vi "KH Control.vi"(6 "Radio Buttons":T1(radio), 8 "error in":errorcluster, 11 "Channel Setting":T7=[{"Channel"=enum."Channel 1", "Gain"=enum."10x", "Shunt Resistor"=enum."Open", "Input Config"=enum."Ground"}, {"Channel"=enum."Channel 2", "Gain"=enum."10x", "Shunt Resistor"=enum."Open", "Input Config"=enum."Ground"}, {"Channel"=enum."Channel 3", "Gain"=enum."10x", "Shunt Resistor"=enum."Open", "Input Config"=enum."Ground"}, {"Channel"=enum."Channel 4", "Gain"=enum."10x", "Shunt Resistor"=enum."Open", "Input Config"=enum."Ground"}, {"Channel"=enum."Channel 5", "Gain"=enum."10x", "Shunt Resistor"=enum."Open", "Input Config"=enum."Ground"}, {"Channel"=enum."Channel 6", "Gain"=enum."10x", "Shunt Resistor"=enum."Open", "Input Config"=enum."Ground"}, {"Channel"=enum."Channel 7", "Gain"=enum."10x", "Shunt Resistor"=enum."Open", "Input Config"=enum."Ground"}, {"Channel"=enum."Channel 8", "Gain"=enum."10x", "Shunt Resistor"=enum."Open", "Input Config"=enum."Ground"}]) -> (0 "error out":errorcluster={"status"=FALSE, "code"=1073676294, "source"="VISA Read in KH7008.lvclass:KH7008 COM.vi->KH7008.lvclass:KH7008 Set All.vi->KH7008.lvclass:KH Control.vi"}, 3 "Channel Settings Used":T2[](array[typedef])=[{"Channel"=enum."Channel 1", "Gain"=enum."10x", "Shunt Resistor"=enum."Open", "Input Config"=enum."Ground"}, {"Channel"=enum."Channel 2", "Gain"=enum."10x", "Shunt Resistor"=enum."Open", "Input Config"=enum."Ground"}, {"Channel"=enum."Channel 3", "Gain"=enum."10x", "Shunt Resistor"=enum."Open", "Input Config"=enum."Ground"}, {"Channel"=enum."Channel 4", "Gain"=enum."10x", "Shunt Resistor"=enum."Open", "Input Config"=enum."Ground"}, {"Channel"=enum."Channel 5", "Gain"=enum."10x", "Shunt Resistor"=enum."Open", "Input Config"=enum."Ground"}, {"Channel"=enum."Channel 6", "Gain"=enum."10x", "Shunt Resistor"=enum."Open", "Input Config"=enum."Ground"}, {"Channel"=enum."Channel 7", "Gain"=enum."10x", "Shunt Resistor"=enum."Open", "Input Config"=enum."Ground"}, {"Channel"=enum."Channel 8", "Gain"=enum."10x", "Shunt Resistor"=enum."Open", "Input Config"=enum."Ground"}])   [LabVIEW 2016, in "KH7008.lvclass"]
uses:
  KH7008.lvclass
  typedefs/KH_control_array.ctl
  typedefs/KH_control.ctl
  typedefs/Channel-Enum.ctl
  typedefs/Gain-Enum.ctl
  typedefs/Shunt-Enum.ctl
  typedefs/Input Configuration-Enum.ctl
  typedefs/SetAll-Cluster.ctl
  typedefs/Filter-Enum.ctl
  typedefs/Coupling-Enum.ctl
  <vilib>/MakerHub/Toolbox/LMH-Toolbox.lvlib
panel:
  in  "VISA Refnum in":refnum<visa-resource-name>="COM3"
  # "Measure Current: Current, Shunt Resistor: 50kOhm\nMeasure Voltage: Voltage, Shunt Resistor: Open\nApplying Gate: Current, Shunt Resistor: 50kOhm\n                      Open all the unused gate\n\n1. Create a copy of drivers under C:\\Krohn-Hite 7008\\Drivers if there is none. \n2. In device manager browse the driver for Krohn-Hite \n\nWarning: repeated channels will cause false reading in the lock-in"
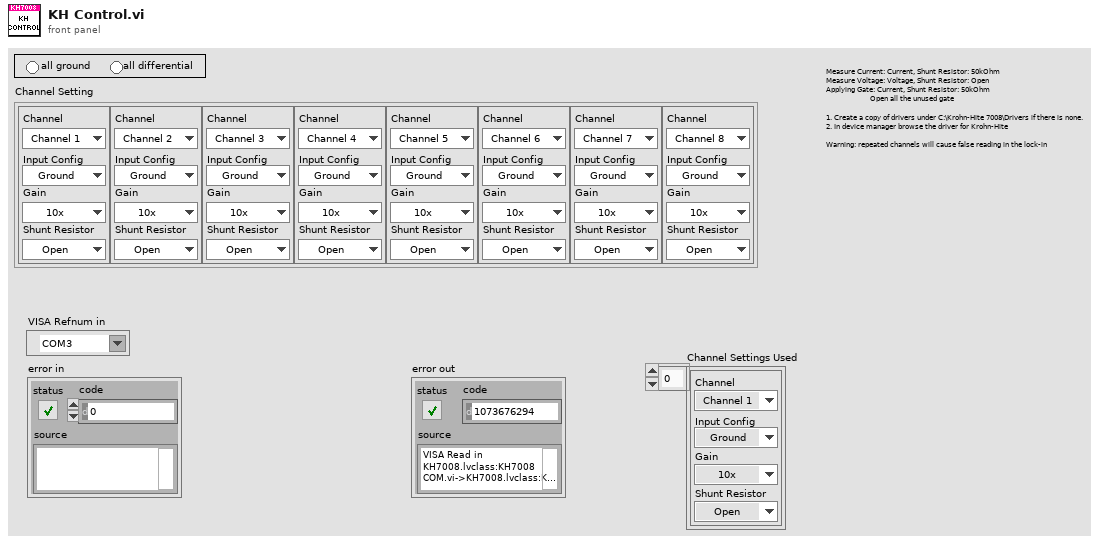
[diagram p1: front panel]
types:
  T1 = enum32{"No Selection", "all ground", "all differential"}
  T2 = typedef "KH7008.lvclass/KH_control.ctl" = cluster{"Channel":T3, "Gain":T4, "Shunt Resistor":T5, "Input Config":T6}
  T3 = typedef "KH7008.lvclass/Channel-Enum.ctl" = enum16{"Channel 1", "Channel 2", "Channel 3", "Channel 4", "Channel 5", "Channel 6", "Channel 7", "Channel 8"}
  T4 = typedef "KH7008.lvclass/Gain-Enum.ctl" = enum16{"1x", "10x", "100x", "1000x"}
  T5 = typedef "KH7008.lvclass/Shunt-Enum.ctl" = enum16{"Open", "50 Ohms", "500 Ohms", "5k Ohms", "50k Ohms"}
  T6 = typedef "KH7008.lvclass/Input Configuration-Enum.ctl" = enum16{"Ground", "SE+ (-gnd)", "SE- (+gnd)", "Differential"}
  T7 = typedef "KH7008.lvclass/KH_control_array.ctl" = T2[]
  T8 = typedef "KH7008.lvclass/Coupling-Enum.ctl" = enum16{"AC", "DC"}
  T9 = typedef "KH7008.lvclass/Filter-Enum.ctl" = enum16{"OFF", "ON"}
  T10 = typedef "KH7008.lvclass/SetAll-Cluster.ctl" = cluster{"Channel":T3, "Gain":T4, "Bandwidth Filter":T9, "Shunt Resistor":T5, "Coupling":T8, "Input Configuration":T6}
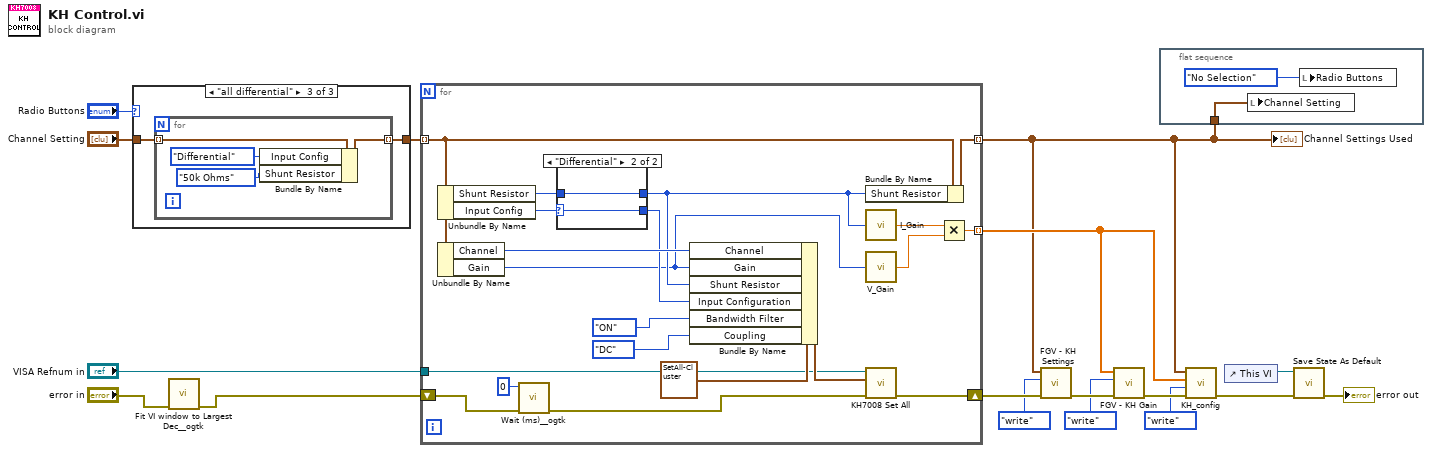
[diagram p0: block diagram]
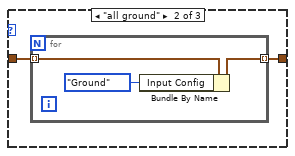
[diagram p3: hidden frame]
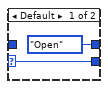
[diagram p4: hidden frame]
diagram:
  n1 = case shown="\"all differential\"" "Radio Buttons" {
    tunnel: [w18 w20 w25] -> w8
    tunnel: "Channel Setting" -> [w18 w19 w24]
    frame "No Selection", Default {
    }
    frame "all ground" {
      n2 = for {
        tunnel: w19 -> [w23] mode=indexing
        tunnel: [w22] -> w20 mode=indexing
        n3 = Bundle By Name(cluster=w23, "Input Config"=Input_Configuration-Enum."Ground") -> (w22:T2)
      }
    }
    frame "all differential" {
      n4 = for {
        tunnel: w24 -> [w29] mode=indexing
        tunnel: [w28] -> w25 mode=indexing
        n5 = Bundle By Name(cluster=w29, "Input Config"=Input_Configuration-Enum."Differential", "Shunt Resistor"=Shunt-Enum."50k Ohms") -> (w28:T2)
      }
    }
  }
  n6 = call <userlib>:"Fit VI window to Largest Dec__ogtk.vi"("error in (no error)"="error in") -> ("error out"=w3:errorcluster)  [unwired: 5 in, 1 out]
  n7 = for {
    tunnel: w8 -> [w34] mode=indexing
    tunnel: [w49] -> w5 mode=indexing
    shift-right: [w47] -> w13
    shift-left: w3 -> [w48]
    tunnel: [w41] -> w1 mode=indexing
    tunnel: "VISA Refnum in" -> [w40]
    n8 = Unbundle By Name(w34) -> ("Shunt Resistor"=w36:T5, "Input Config"=w35:T6)
    n9 = Unbundle By Name(w34) -> ("Channel"=w39:T3, "Gain"=w30:T4)
    n10 = call <userlib>:"Wait (ms)__ogtk.vi"("error in (no error)"=w48, "milliseconds to wait"=u32 0) -> ("error out"=w46:errorcluster)  [unwired: 8 in, 1 out]
    n11 = case shown="\"Differential\"" w35 {
      selector: w35 -> [w50 w52]
      tunnel: [Shunt-Enum."Open" ("f") w53] -> w33
      tunnel: w36 -> [_ w53]
      tunnel: [w50 w52] -> w31
      frame Default {
      }
      frame "Differential" {
      }
    }
    n12 = Bundle By Name(cluster=T10 {"Channel"=enum."Channel 2", "Gain"=enum."10x", "Bandwidth Filter"=enum."ON", "Shunt Resistor"=enum."50 Ohms", "Coupling"=enum."DC", "Input Configuration"=enum."Differential"} ("Set All"), "Channel"=w39, "Gain"=w30, "Shunt Resistor"=w33, "Input Configuration"=w31, "Bandwidth Filter"=Filter-Enum."ON", "Coupling"=Coupling-Enum."DC") -> (w43:T10)
    n13 = Bundle By Name(cluster=w34, "Shunt Resistor"=w33) -> (w41:T2)
    n14 = call "I_Gain.vi"("Shunt Resistor"=w33) -> ("Gain (V/A)"=w42:dbl)
    n15 = call "V_Gain.vi"("Gain"=w30) -> ("Gain (x)"=w32:dbl)
    n16 = call "KH7008 Set All.vi"("error in (no error)"=w46, "Set All"=w43, "VISA Refnum in"=w40) -> ("error out"=w47:errorcluster)  [unwired: 8 in]
    n17 = Multiply(x=w42, y=w32) -> (x*y=w49:dbl)
  }
  "Channel Settings Used" <- w1
  n18 = call "FGV - KH Settings.vi"("error in"=w13, "Function"=enum16{"write", "read"}."write", "Channel Setting"=w1) -> ("error out"=w14:errorcluster)  [unwired: 3 in, 1 out]
  n19 = call "FGV - KH Gain.vi"("error in"=w14, "Function"=enum16{"write", "read"}."write", "Gains"=w5) -> ("error out"=w15:errorcluster)  [unwired: 3 in, 1 out]
  n20 = flat-sequence {
    tunnel: w1 -> [w55]
    frame #0 {
      n21 = local write "Channel Setting"(w55) -> ()
      n22 = local write "Radio Buttons"(T1."No Selection" ("Radio Buttons 2")) -> ()
    }
  }
  n23 = call "KH_config.vi"("Error In"=w15, "Function"=enum16{"write", "read"}."write", "Gains"=w5, "Channel Setting"=w1) -> ("Error Out"=w16:errorcluster)  [unwired: 5 in, 2 out]
  n24 = control-ref of="This VI"() -> (w11:refnum<vi>)
  n25 = call <vilib>:"Save State As Default.vi"("Error In"=w16, "Target VI"=w11) -> ("Error Out"=→"error out":errorcluster)  [unwired: 8 in, 1 out]
